vi "offline version.vi"(7 "error in":errorcluster) -> (21 "Calibrated Matches (Pattern Matching 1)":T3(array[cluster]) {"Bounding Box"."y" format="%.2f"; "Bounding Box"."x" format="%.2f"; "Position"."y" format="%.2f"; "Position"."x" format="%.2f"; "Score" format="%.2f"; "Scale" format="%.2f"; "Angle" format="%.2f"}, 22 "Number of Matches (Pattern Matching 1)":i32, 27 "error out":errorcluster)   [LabVIEW 2013]
uses:
  <vilib>/vision/NI_Vision_Development_Module.lvlib
panel:
  in  "Font, Size & Style":T1={"Desired Font (Application)"=enum."Application Font", "[User-specified Font]"={"Font Name"="", "Size"=12, "Strikeout?"=FALSE, "Italic?"=FALSE, "Underline?"=FALSE, "Outline?"=FALSE, "Shadow?"=FALSE, "Bold?"=FALSE, "Rotation Angle"=0.0}, "Horizontal Alignment"=0, "Vertical Alignment"=0} {"Vertical Alignment" items=["Bottom", "Top", "Baseline"]; "Horizontal Alignment" items=["Left", "Center", "Right"]; "[User-specified Font]"."Rotation Angle" format="%.2f"}
  out "Mean Value":sgl
  out "Image Out 2":T2(plugin-control)
  out "output cluster":cluster{sgl, sgl, sgl, sgl, i32}
  out "Position":cluster{"x":sgl, "y":sgl}
  out "Image Out":T2(plugin-control)
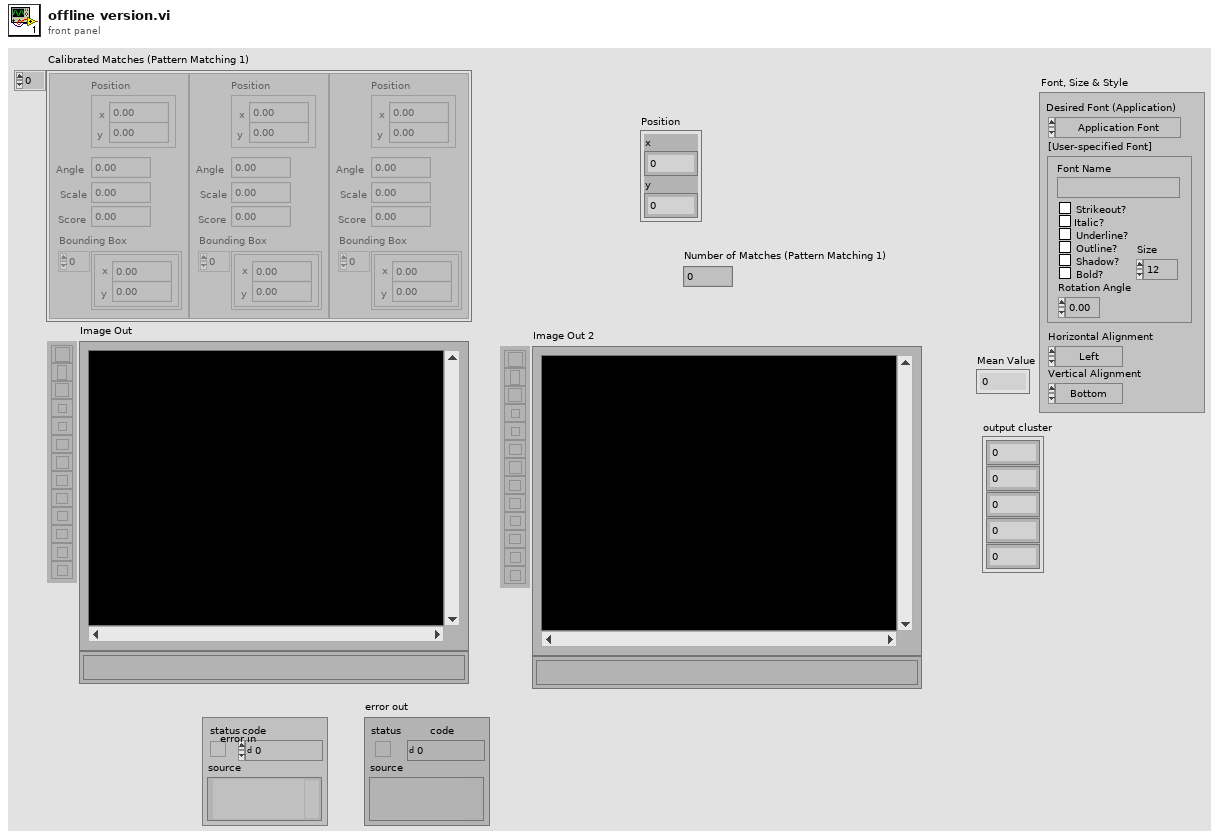
[diagram p1: front panel]
types:
  T1 = cluster{"Desired Font (Application)":enum16{"User-specified Font", "Application Font", "System Font", "Dialog Font"}, "[User-specified Font]":cluster{"Font Name":string, "Size":i16, "Strikeout?":bool, "Italic?":bool, "Underline?":bool, "Outline?":bool, "Shadow?":bool, "Bold?":bool, "Rotation Angle":dbl}, "Horizontal Alignment":i16, "Vertical Alignment":i16}
  T2 = typedef "IMAQ Image.ctl" = refnum<image>
  T3 = cluster{"Position":cluster{"x":sgl, "y":sgl}, "Angle":sgl, "Scale":sgl, "Score":sgl, "Bounding Box":cluster{"x":sgl, "y":sgl}[]}[]
  T4 = cluster{"Number of Matches Requested":i32, "Minimum Match Score":sgl, "Angle Ranges":cluster{"Start Angle":sgl, "End Angle":sgl}[]}
  T5 = cluster{"Global Rectangle":i32[], "Contours":cluster{"ID":enum32{"External", "Internal"}, "Type":u32, "Coordinates":i32[]}[]}
  T6 = typedef "IMAQ Rectangle" = cluster{"Left":i32, "Top":i32, "Right":i32, "Bottom":i32, "Rotation":dbl}
  T7 = typedef "Image Type" = u32
  T8 = cluster{"Minimal Value":sgl, "Maximal Value":sgl, "Mean Value":sgl, "Standard  Variation":sgl, "Area (pixels)":i32}
  T9 = cluster{"Position":cluster{"x":sgl, "y":sgl}, "Angle":sgl, "Scale":sgl, "Score":sgl, "Bounding Box":cluster{"x":sgl, "y":sgl}[]}
  T10 = typedef "ROI Descriptor" = cluster{"Global Rectangle":i32[], "Contours":cluster{"ID":enum32{"External", "Internal"}, "Type":u32, "Coordinates":i32[]}[]}
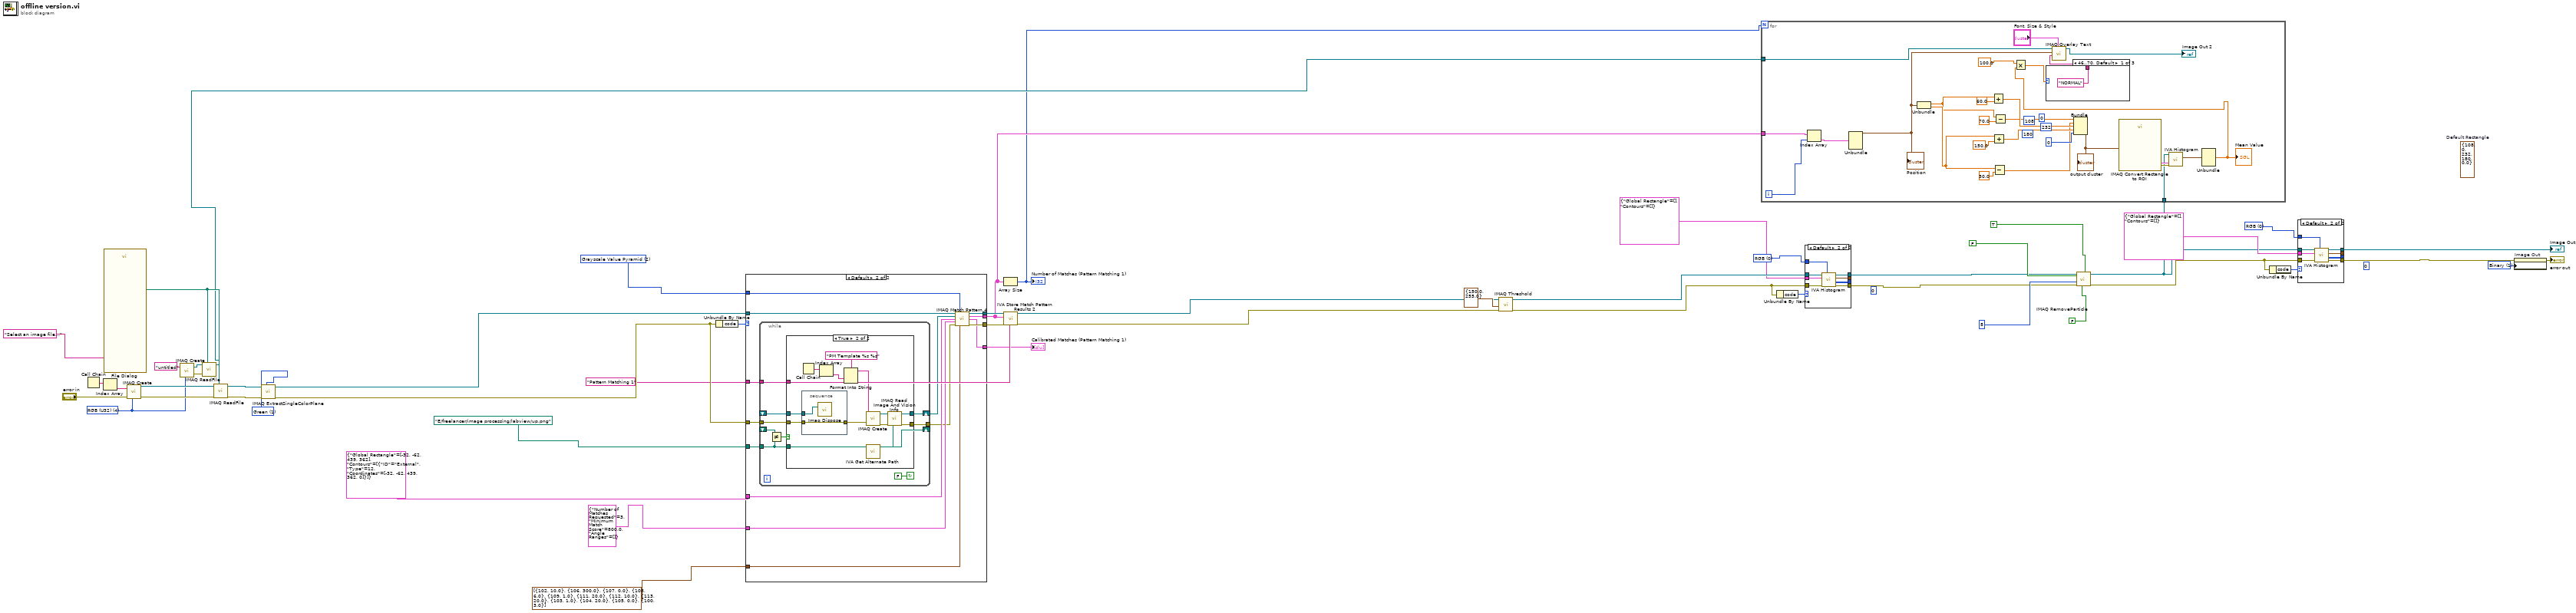
[diagram p0: block diagram]
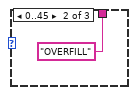
[diagram p2: hidden frame]
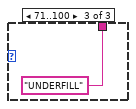
[diagram p3: hidden frame]
diagram:
  w48 = 1 items=["Red", "Green", "Blue", "Hue", "Saturation", "Luminance", "Value", "Intensity"] ("Color Plane (Color Plane Extraction 1)")
  w41 = 2 items=["All", "Low Discrepancy Sampling", "Grayscale Value Pyramid", "Gradients Pyramid"] ("Algorithm (Pattern Matching 1)")
  w24 = u16 0 items=["RGB", "HSL", "HSV", "HSI"] ("Color Mode (Histogram 1)")
  w32 = u16 0 items=["RGB", "HSL", "HSV", "HSI"] ("Color Mode (Histogram 2)")
  (unwired) T6 {"Left"=108, "Top"=0, "Right"=232, "Bottom"=180, "Rotation"=0.0}  # Default Rectangle
  w21 = u32 1 items=["Grayscale", "Binary", "Gradient", "Rainbow", "Temperature", "User Defined"] ("Palette")
  (unwired) u8 0 ("Y Scale.Mapping Mode")
  (unwired) u8 0 ("Y Scale.Mapping Mode")
  w37 = "Pattern Matching 1" ("Step Name")
  w5 = T7 4 items=["Grayscale (U8)", "Grayscale (I16)", "Grayscale (SGL)", "Complex (CSG)", "RGB (U32)", "HSL (U32)", "RGB (U64)", "Grayscale (U16)"] ("Image Type")
  n1 = Call Chain() -> (call chain=w49:string[])
  n2 = Index Array(array=w49) -> (element=w10:string)  [unwired: 1 in]
  n3 = call "File Dialog"("prompt"="Select an image file...") -> ("selected path"=w6:path)  [unwired: 6 in, 8 out]
  n4 = call "IMAQ Create"("Image Name"=w10, "Image Type"=w5, "error in (no error)"="error in") -> ("New Image"=w11:T2, "error out"=w51:errorcluster)  [unwired: 1 in, 1 out]
  n5 = call "IMAQ Create"("Image Name"="untitled", "Image Type"=w5) -> ("New Image"=w7:T2, "error out"=w8:errorcluster)  [unwired: 2 in, 1 out]
  n6 = call "IMAQ ReadFile"("File Path"=w6, "error in (no error)"=w8, "Image"=w7) -> ("Image Out"=w4:T2)  [unwired: 2 in, 6 out]
  n7 = call "IMAQ ReadFile"("File Path"=w6, "error in (no error)"=w51, "Image"=w11) -> ("error out"=w52:errorcluster, "Image Out"=w12:T2)  [unwired: 2 in, 5 out]
  n8 = call "IMAQ ExtractSingleColorPlane"("Color Plane"=w48, "error in (no error)"=w52, "Image Src"=w12) -> ("error out"=w47:errorcluster, "Image Dst Out"=w45:T2)  [unwired: 1 in, 6 out]
  n9 = Unbundle By Name(w47) -> ("code"=w42:i32)
  n10 = case shown="Default" w42 {
    tunnel: path "E:/freelancer/image processing/labview/up.png" ("Template File Path (Pattern Matching 1)") -> [_ w67]
    tunnel: w47 -> [_ w66]
    tunnel: w45 -> [w53 w61]
    tunnel: [_ w62] -> w44
    tunnel: [_ w63] -> w13
    tunnel: [w53 w60] -> w43
    tunnel: w37 -> [_ w65]
    tunnel: w41 -> [_ w59]
    tunnel: T5 {"Global Rectangle"=[-32, -62, 439, 362], "Contours"=[{"ID"=enum."External", "Type"=12, "Coordinates"=[-32, -62, 439, 362, 0]}]} ("ROI Descriptor (Pattern Matching 1)") -> [_ w58]
    tunnel: T4 {"Number of Matches Requested"=3, "Minimum Match Score"=800.0, "Angle Ranges"=[]} ("Parameters (Pattern Matching 1)") -> [_ w57]
    tunnel: cluster{"Item":u16, "Value":dbl}[] [{"Item"=102, "Value"=10.0}, {"Item"=106, "Value"=300.0}, {"Item"=107, "Value"=0.0}, {"Item"=108, "Value"=6.0}, {"Item"=109, "Value"=1.0}, {"Item"=111, "Value"=20.0}, {"Item"=112, "Value"=10.0}, {"Item"=113, "Value"=20.0}, {"Item"=103, "Value"=1.0}, {"Item"=104, "Value"=20.0}, {"Item"=105, "Value"=0.0}, {"Item"=100, "Value"=3.0}] ("Advanced Options (Pattern Matching 1)") -> [_ w55]
    tunnel: [_ w54] -> w36
    frame -1074396199, -1074396198 {
      # "Discard Coordinate System Error"
    }
    frame Default {
      n11 = while {
        shift-right: [w76] -> w64
        shift-left: _ -> [w75]
        tunnel: [w73] -> w56
        tunnel: w66 -> [w72]
        tunnel: w67 -> [w69]
        tunnel: w65 -> [w71]
        shift-right: [w69] -> _
        shift-left: _ -> [w70]
        stop <- FALSE continue-if-true
        n12 = Not Equal?(x=w70, y=w69) -> (x != y?=w68:bool)
        n13 = case shown="True" w68 {
          tunnel: [w78 w90] -> w76
          tunnel: w75 -> [w78 w81]
          tunnel: [w77 w87] -> w73
          tunnel: w72 -> [w77 w80]
          tunnel: w69 -> [_ w83]
          tunnel: w71 -> [_ w84]
          frame False {
          }
          frame True {
            n14 = stacked-sequence {
              tunnel: w81 -> [w94]
              tunnel: w80 -> [w93]
              tunnel: [w93] -> w79
              frame #0 {
                n15 = call "Imaq Dispose"("Image"=w94) -> ()  [unwired: 2 in, 4 out]
              }
            }
            n16 = Call Chain() -> (call chain=w86:string[])
            n17 = Index Array(array=w86) -> (element=w85:string)  [unwired: 1 in]
            n18 = Format Into String(format string="PM Template %s %s" ("Image Name"), w85, w84) -> (resulting string=w92:string)  [unwired: 2 in, 1 out]
            n19 = call "IMAQ Create"("Image Name"=w92, "error in (no error)"=w79) -> ("New Image"=w89:T2, "error out"=w88:errorcluster)  [unwired: 2 in, 1 out]
            n20 = call <vilib>:"IVA Get Alternate Path.vi"("Path In"=w83) -> ("Path Out"=w82:path)  [unwired: 10 out]
            n21 = call "IMAQ Read Image And Vision Info"("File Path"=w82, "error in (no error)"=w88, "Image"=w89) -> ("error out"=w87:errorcluster, "Image Out"=w90:T2)  [unwired: 1 in, 6 out]
          }
        }
      }
      n22 = call "IMAQ Match Pattern 4"("Image"=w61, "Algorithm"=w59, "Template Image"=w64, "ROI Descriptor"=w58, "Parameters"=w57, "error in (no error)"=w56, "Advanced Options"=w55) -> ("Image (duplicate)"=w60:T2, "Matches (pixel)"=w63:T3, "Matches (real-world)"=w54:T3, "error out"=w62:errorcluster)  [unwired: 4 in, 1 out]
    }
  }
  "Calibrated Matches (Pattern Matching 1)" <- w36
  n23 = Array Size(array=w13) -> (size(s)=w3:i32)
  "Number of Matches (Pattern Matching 1)" <- w3
  n24 = call <vilib>:"IVA Store Match Pattern Results 2.vi"("Step Name"=w37, "error in (no error)"=w44, "Matches (pixel)"=w13, "Image in"=w43) -> ("error out"=w17:errorcluster, "Image dup"=w18:T2)  [unwired: 2 in, 4 out]
  n25 = call "IMAQ Threshold"("error in (no error)"=w17, "Range"=cluster{"Lower value":sgl, "Upper value":sgl} {"Lower value"=150.0, "Upper value"=255.0} ("Range (Threshold 1)"), "Image Src"=w18) -> ("error out"=w34:errorcluster, "Image Dst Out"=w33:T2)  [unwired: 3 in, 4 out]
  n26 = Unbundle By Name(w34) -> ("code"=w30:i32)
  n27 = case shown="Default" w30 {
    tunnel: w34 -> [_ w103]
    tunnel: w33 -> [w95 w102]
    tunnel: [_ w101] -> _
    tunnel: [_ w100] -> w2
    tunnel: w32 -> [_ w99]
    tunnel: [_ w98] -> _
    tunnel: T5 {"Global Rectangle"=[], "Contours"=[]} ("ROI Descriptor (Histogram 2)") -> [_ w97]
    tunnel: [w95 w96] -> w25
    frame -1074396199, -1074396198 {
      # "Discard\nCoordinate\nSystem\nError"
    }
    frame Default {
      n28 = call <vilib>:"IVA Histogram.vi"("Color Mode"=w99, "error in (no error)"=w103, "ROI Descriptor"=w97, "Image In"=w102) -> ("error out"=w100:errorcluster, "Histograms"=w98:u32[][], "Statistics"=w101:T8, "Image Out"=w96:T2)  [unwired: 4 out]
    }
  }
  n29 = call "IMAQ RemoveParticle"("Connectivity 4/8 (8)"=TRUE ("Connectivity 4/8 (8) (Adv. Morphology 1)"), "Low Pass/High Pass (Low)"=FALSE ("Low Pass/High Pass (Low) (Adv. Morphology 1)"), "Square/Hexa (Square)"=FALSE ("Square/Hexa (Square) (Adv. Morphology 1)"), "error in (no error)"=w2, "Number of Erosion"=8 ("Number of Erosion (Adv. Morphology 1)"), "Image Src"=w25) -> ("error out"=w16:errorcluster, "Image Dst Out"=w14:T2)  [unwired: 1 in, 3 out]
  n30 = for {
    N: w3 -> [_]
    tunnel: w14 -> [w128]
    tunnel: w13 -> [w126]
    tunnel: w4 -> [w111]
    i -> [w105]
    (unwired) 180
    (unwired) 232
    (unwired) 108
    (unwired) 0
    n31 = Index Array(array=w126, index=w105) -> (element=w127:T9)
    n32 = Unbundle(w127) -> ("Position"=w113:cluster{"x":sgl, "y":sgl})  [unwired: 4 out]
    "Position" <- w113
    n33 = Unbundle(w113) -> ("x"=w118:sgl, "y"=w123:sgl)
    n34 = Add(x=w118, y=sgl 60.0) -> (x+y=w117:sgl)
    n35 = Add(x=w123, y=sgl 150.0) -> (x+y=w116:sgl)
    n36 = Subtract(x=w123, y=sgl 30.0) -> (x-y=w115:sgl)
    n37 = Subtract(x=w118, y=sgl 70.0) -> (x-y=w114:sgl)
    n38 = Bundle(w114, w115, w117, w116, 0) -> (w125:cluster{sgl, sgl, sgl, sgl, i32})  [unwired: 1 in]
    "output cluster" <- w125
    n39 = call "IMAQ Convert Rectangle to ROI"("Rectangle"=w125) -> ("error out"=w130:errorcluster, "ROI Descriptor"=w129:T10)  [unwired: 8 in]
    n40 = call <vilib>:"IVA Histogram.vi"("error in (no error)"=w130, "ROI Descriptor"=w129, "Image In"=w128) -> ("Statistics"=w112:T8)  [unwired: 1 in, 7 out]
    n41 = Unbundle(w112) -> ("Mean Value"=w108:sgl)  [unwired: 4 out]
    "Mean Value" <- w108
    n42 = Multiply(x=sgl 100.0 ("y"), y=w108) -> (x*y=w106:sgl)
    n43 = case shown="46..70, Default" w106 {
      tunnel: ["NORMAL" ("String") "OVERFILL" ("String") "UNDERFILL" ("String")] -> w110
      frame 46..70, Default {
      }
      frame 0..45 {
      }
      frame 71..100 {
      }
    }
    n44 = call "IMAQ Overlay Text"("Font, Size & Style"="Font, Size & Style", "String"=w110, "Origin"=w113, "Image"=w111) -> ("Image Out"=→"Image Out 2":T2)  [unwired: 6 in, 1 out]
  }
  n45 = Unbundle By Name(w16) -> ("code"=w22:i32)
  n46 = case shown="Default" w22 {
    tunnel: w16 -> [_ w142]
    tunnel: w14 -> [w134 w141]
    tunnel: [_ w140] -> _
    tunnel: [_ w139] -> w1
    tunnel: w24 -> [_ w138]
    tunnel: [_ w137] -> _
    tunnel: T5 {"Global Rectangle"=[], "Contours"=[]} ("ROI Descriptor (Histogram 1)") -> [_ w136]
    tunnel: [w134 w135] -> w19
    frame -1074396199, -1074396198 {
      # "Discard\nCoordinate\nSystem\nError"
    }
    frame Default {
      n47 = call <vilib>:"IVA Histogram.vi"("Color Mode"=w138, "error in (no error)"=w142, "ROI Descriptor"=w136, "Image In"=w141) -> ("error out"=w139:errorcluster, "Histograms"=w137:u32[][], "Statistics"=w140:T8, "Image Out"=w135:T2)  [unwired: 4 out]
    }
  }
  "Image Out" <- w19
  n48 = property on="Image Out" class="ImageControl"(error in=w1, "Palette:Palette Type"=w21) -> (error out=→"error out":errorcluster)  [unwired: 1 in, 1 out]
